vi "Initialize_movie.vi"(9 "Frames Per Second":u32=30, 11 "Ch#":string=" 1.avi") -> (3 "AVI Refnum":T1)   [LabVIEW 2016]
uses:
  <vilib>/vision/Avi.llb/IMAQ AVI2 Refnum.ctl
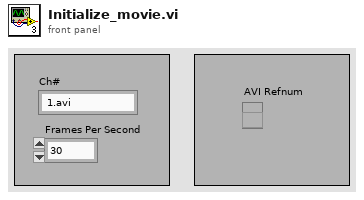
[diagram p1: front panel]
types:
  T1 = typedef "IMAQ AVI2 Refnum.ctl" = refnum<k20>
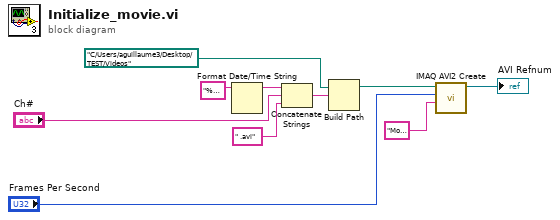
[diagram p0: block diagram]
diagram:
  n1 = Format Date/Time String(time format string (%c)="%H %M %S") -> (date/time string=w10:string)  [unwired: 2 in]
  n2 = Concatenate Strings(w10, "Ch#", " .avi" ("initial string")) -> (w9:string)
  n3 = Build Path(base path=path "C:/Users/aguillaume3/Desktop/TEST/Videos", name or relative path=w9) -> (appended path=w3:path)
  n4 = call "IMAQ AVI2 Create"("Codec"="Motion JPEG (NI Vision)", "Frames Per Second"="Frames Per Second", "AVI Path"=w3) -> ("AVI Refnum"=→"AVI Refnum":T1)  [unwired: 7 in, 1 out]
